vi "ReadProgramData.vi"(8 "error in (no error)":errorcluster, 11 "file path (dialog if empty)":path) -> (0 "error out":errorcluster, 1 "Number of steps":i32, 2 "Program data":dbl[][](array[numeric]), 3 "Program":string[][](table), 5 "Est. time":dbl)   [LabVIEW 2013]
uses:
  controls/ProgramColumn.ctl
  <vilib>/Utility/file.llb/Read From Spreadsheet File (string).vi
  <vilib>/Utility/file.llb/Read From Spreadsheet File (DBL).vi
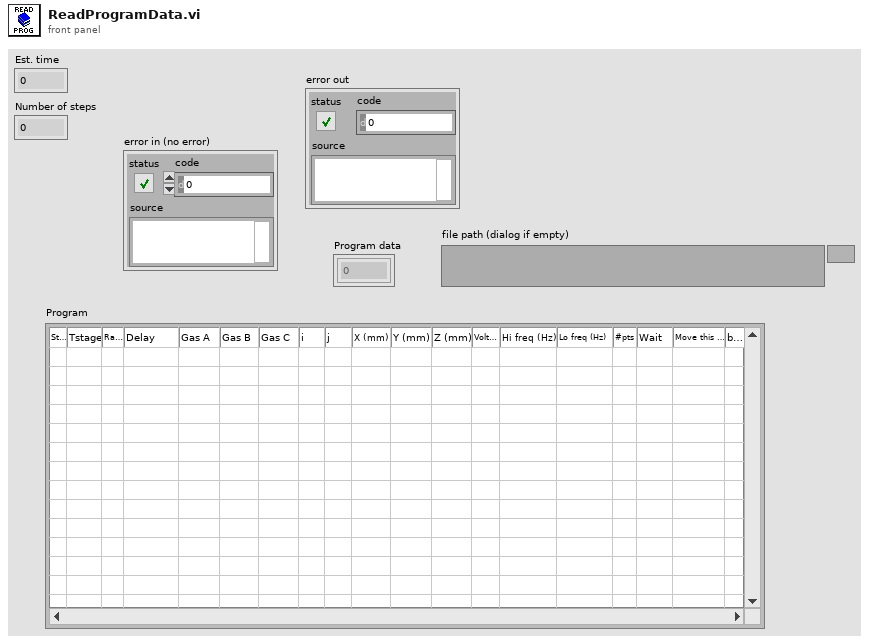
[diagram p1: front panel]
types:
  T1 = typedef "ProgramColumn.ctl" = enum16{"Run Number", "Stage Temperature", "Ramp Rate", "Wait", "Gas A", "Gas B", "Gas C", "Row index I", "Column index J", "X position", "Y position", "Z position", "Voltage", "Highest frequency", "Lowest frequency", "Number of freq pts", "Delay", "Move this step?", "bias(V)"}
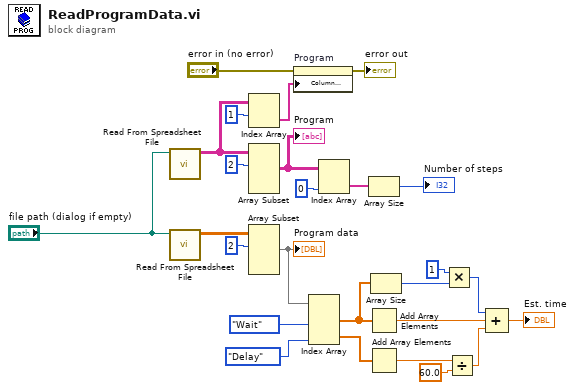
[diagram p0: block diagram]
diagram:
  n1 = call-poly <vilib>:"Read From Spreadsheet File.vi"("file path (dialog if empty)"="file path (dialog if empty)") -> ("all rows"=w26:string[][])  [unwired: 6 in, 4 out]
  n2 = call-poly <vilib>:"Read From Spreadsheet File.vi"("file path (dialog if empty)"="file path (dialog if empty)") -> ("all rows"=w22:dbl[][])  [unwired: 6 in, 4 out]
  n3 = Index Array(array=w26, index (row)=1) -> (element=w24:string[])  [unwired: 1 in]
  n4 = Array Subset(array=w26, index (row)=2 ("index")) -> (w20:string[][])  [unwired: 3 in]
  "Program" <- w20
  n5 = Array Subset(array=w22, index (row)=2 ("index")) -> (w17:dbl[][])  [unwired: 3 in]
  "Program data" <- w17
  n6 = property on="Program" class="Tbl (strict)"(error in="error in (no error)", "Column Headers[]"=w24) -> (error out=→"error out":errorcluster)  [unwired: 1 in, 1 out]
  n7 = Index Array(array=w17, index (col) #1=ProgramColumn."Wait" ("Enum"), index (col) #2=ProgramColumn."Delay" ("Enum")) -> (element #1=w11:dbl[], element #2=w14:dbl[])  [unwired: 2 in]
  n8 = Index Array(array=w20, index (col)=0 ("index (row)")) -> (element=w19:string[])  [unwired: 1 in]
  n9 = Array Size(array=w19) -> (size(s)=→"Number of steps":i32)
  n10 = Add Array Elements(numeric array=w11) -> (sum=w7:dbl)
  n11 = Add Array Elements(numeric array=w14) -> (sum=w13:dbl)
  n12 = Array Size(array=w11) -> (size(s)=w10:i32)
  n13 = Multiply(x=1, y=w10) -> (x*y=w8:i32)
  n14 = Divide(x=w13, y=60.0) -> (x/y=w6:dbl)
  n15 = Compound Arithmetic op=ADD(w8, w7, w6) -> (→"Est. time":dbl)
